vi "Periodic Tasks.vi"(8 "error in":errorcluster) -> ()   [LabVIEW 2013]
doc: "This VI runs in parallel to other tasks. It can contain as many user-defined periodic loops as you need. These can carry out PID or other sorts of timed response."
uses:
  PressureSensorAction.ctl
  <vilib>/Rock Robotics/SystemInterfaces/Utilities/FPGA_UtilitiesLED Source.ctl
  <vilib>/Rock Robotics/SystemInterfaces/Utilities/FPGA_UtilitiesLED State.ctl
  PassType.ctl
  PassState.ctl
  <vilib>/Rock Robotics/WPI/Compressor/WPI_CompressorGetSetRefNum.vi
  Robot Global Data.vi
panel:
  out "Pressure Sensor Iterations":i32
  out "Pressure Sensor Loop Time":u32
  out "Handler Iterations":i32
  in  "HalfDriveScalar":dbl=0.6
  out "Handler Skipped Data?":bool
  out "Main Loop Time":u32
  out "Handler Loop Time":u32
  out "Drive Loop Time":u32
  out "HandleInputElements":i32
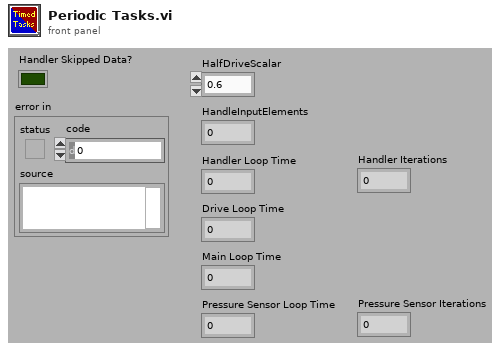
[diagram p1: front panel]
types:
  T1 = typedef "TeleopInstruction.ctl" = cluster{"cDriveLeft":dbl, "cDriveRight":dbl, "cAutoDistance":bool, "cHalfDrive":bool, "cStraightDrive":bool, "cReverseDrive":bool, "cSonicShifter":bool, "cRoller":dbl, "cCollector":dbl, "cServo":dbl, "cPass":bool, "cCatch":bool, "cCollectorWrap":bool, "cShooter":bool, "cClapperIn":bool, "cClapperOut":bool, "cFiringPneumatic":bool, "cKickerPneumatic":bool, "cRollerPneumatic":bool, "TeleopID":i32}
  T2 = typedef "DriveInstruction.ctl" = cluster{"DriveData":T3, "Subsystem":T4, "Action":T5}
  T3 = typedef "DriveData.ctl" = cluster{"cDriveLeft":dbl, "cDriveRight":dbl, "cHalfDrive":bool, "cStraightDrive":bool, "cReverseDrive":bool}
  T4 = typedef "QueueSubsystem.ctl" = enum16{"Drive", "SonicShifter", "Kicker", "FiringPneumatic", "RollerPneumatic", "Clapper", "RollerMotor", "CollectorMotor", "Servo", "ShooterWrapper", "CollectorWrapper", "CatcherWrapper", "AutoDistance", "PassWrapper"}
  T5 = typedef "TankDriveAction.ctl" = enum16{"Init", "LinearDrive", "SetValue", "Disable"}
  T6 = typedef "FPGA_UtilitiesLED State.ctl" = enum16{"Off", "On", "Toggle"}
  T7 = typedef "FPGA_UtilitiesLED Source.ctl" = enum16{"User LED", "FPGA LED"}
  T8 = typedef "PassType.ctl" = enum16{"Ground", "Elevated"}
  T9 = typedef "PassState.ctl" = enum16{"Pass", "Stop"}
  T10 = typedef "QueueInstruction.ctl" = cluster{"Data":variant, "Subsystem":T4, "Action":T11}
  T11 = typedef "QueueAction.ctl" = enum16{"Init", "SetValue", "Disable"}
  T12 = typedef "DoubleSolenoidAction.ctl" = enum16{"Init", "Middle", "In", "Out"}
  T13 = typedef "RollerAction.ctl" = enum16{"Init", "Off", "Forward", "Reverse"}
  T14 = typedef "CollectorWrapAction.ctl" = enum16{"PreCollect", "Collect", "Stop"}
  T15 = typedef "ServoAction.ctl" = enum16{"Init", "SetAngle", "GetAngle", "Lower", "Raise", "Disable"}
  T16 = typedef "ShooterWrapperAction.ctl" = enum16{"Init", "CollectorDown", "CollectorUp"}
  T17 = typedef "CatchAction.ctl" = enum16{"PreCatch", "Catch", "Stop"}
  T18 = typedef "PressureSensorAction.ctl" = enum16{"Init", "ReadValue", "Disable"}
  T19 = typedef "WPI_CompressorDevRef.ctl" = cluster{"DevStatus":errorcluster, "DigitalInputDevRef":T20, "RelayDevRef":T23}
  T20 = typedef "WPI_DigitalInputDevRef.ctl" = cluster{"DevStatus":errorcluster, "DIO Channel":T21, "Digital Module":T22}
  T21 = typedef "FPGA_DIOChannel.ctl" = enum8{"DIO 1", "DIO 2", "DIO 3", "DIO 4", "DIO 5", "DIO 6", "DIO 7", "DIO 8", "DIO 9", "DIO 10", "DIO 11", "DIO 12", "DIO 13", "DIO 14", "Invalid"}
  T22 = typedef "FPGA_TypedefDigitalModule.ctl" = enum16{"Digital Module 1", "Digital Module 2"}
  T23 = typedef "WPI_RelayDevRef.ctl" = cluster{"DevStatus":errorcluster, "Relay Channel":T24, "Digital Module":T22, "Relay Direction":T25}
  T24 = typedef "FPGA_DIORelayChannel.ctl" = enum8{"Relay 1", "Relay 2", "Relay 3", "Relay 4", "Relay 5", "Relay 6", "Relay 7", "Relay 8", "Invalid"}
  T25 = typedef "WPI_RelayDirection.ctl" = enum16{"Both directions", "Forward only", "Reverse only"}
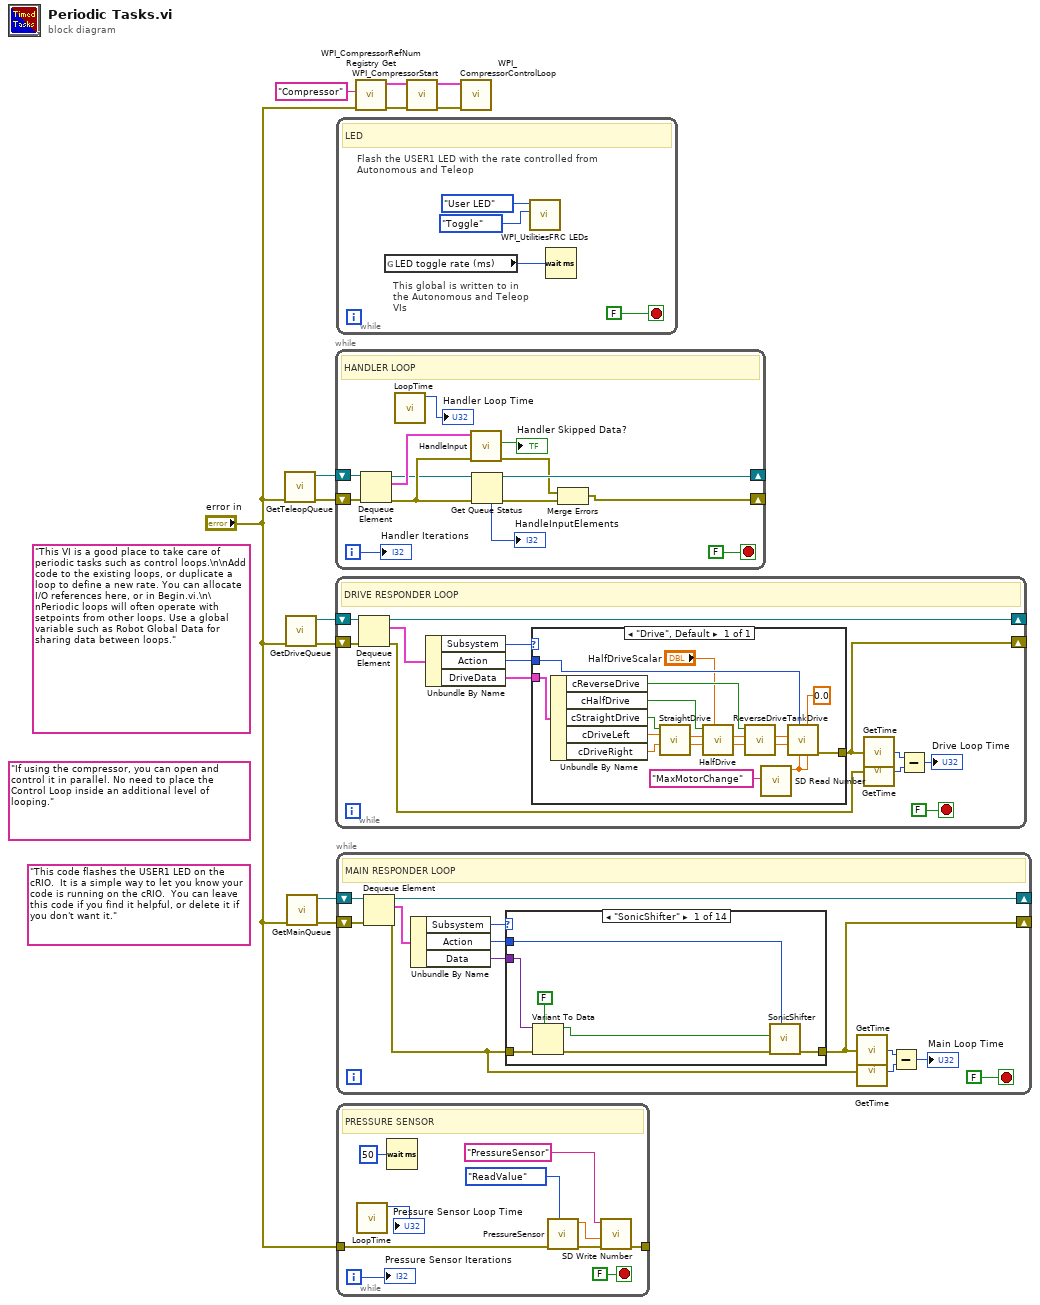
[diagram p0: block diagram]
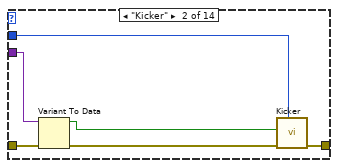
[diagram p2: hidden frame]
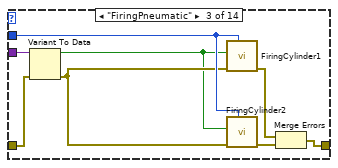
[diagram p3: hidden frame]
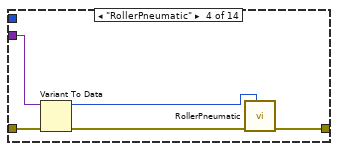
[diagram p4: hidden frame]
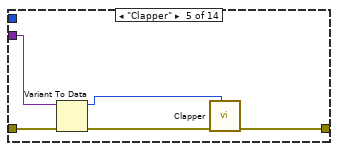
[diagram p5: hidden frame]
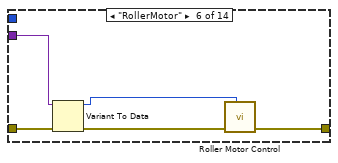
[diagram p6: hidden frame]
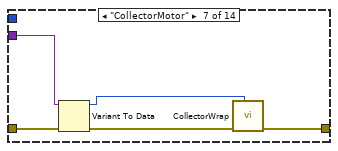
[diagram p7: hidden frame]
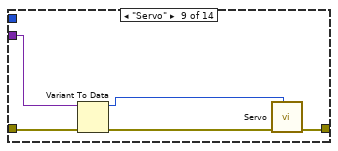
[diagram p9: hidden frame]
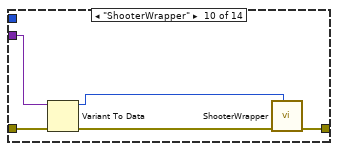
[diagram p10: hidden frame]
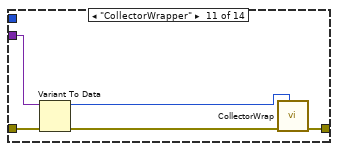
[diagram p11: hidden frame]
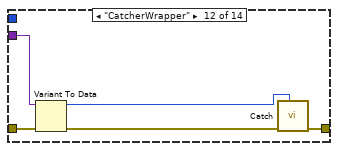
[diagram p12: hidden frame]
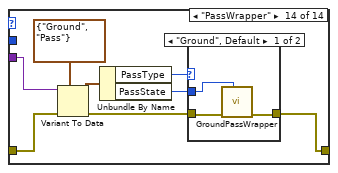
[diagram p14: hidden frame]
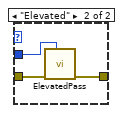
[diagram p15: hidden frame]
diagram:
  (unwired) "If using the compressor, you can open and control it in parallel. No need to place the Control Loop inside an additional level of looping."
  (unwired) "This code flashes the USER1 LED on the cRIO.  It is a simple way to let you know your code is running on the cRIO.  You can leave this code if you find it helpful, or delete it if you don't want it."
  (unwired) "This VI is a good place to take care of periodic tasks such as control loops.\n\nAdd code to the existing loops, or duplicate a loop to define a new rate. You can allocate I/O references here, or in Begin.vi.\n\nPeriodic loops will often operate with setpoints from other loops. Use a global variable such as Robot Global Data for sharing data between loops."
  n1 = call "GetTeleopQueue.vi"("error in (no error)"="error in") -> ("error out"=w6:errorcluster, "queue out"=w7:refnum<queue>)  [unwired: 9 in]
  n2 = call "GetDriveQueue.vi"("error in (no error)"="error in") -> ("error out"=w5:errorcluster, "queue out"=w4:refnum<queue>)  [unwired: 9 in]
  n3 = call "GetMainQueue.vi"("error in (no error)"="error in") -> ("error out"=w2:errorcluster, "queue out"=w3:refnum<queue>)  [unwired: 9 in]
  n4 = while {
    shift-right: [w17] -> _
    shift-left: w6 -> [w26]
    shift-right: [w24] -> _
    shift-left: w7 -> [w25]
    i -> [w13]
    stop <- FALSE stop-if-true
    # "HANDLER LOOP"
    n5 = Dequeue Element(queue=w25, error in (no error)=w26) -> (queue out=w20:refnum<queue>, element=w22:T1, error out=w21:errorcluster)  [unwired: 1 in, 1 out]
    n6 = call "LoopTime.vi"() -> ("LoopTime"=→"Handler Loop Time":u32)  [unwired: 11 in]
    n7 = call "HandleInput.vi"("error in (no error)"=w21, "TeleopInstruction"=w22) -> ("error out"=w18:errorcluster, "SkippedData?"=→"Handler Skipped Data?":bool)  [unwired: 7 in, 1 out]
    n8 = Get Queue Status(queue=w20, error in (no error)=w21) -> (queue out=w24:refnum<queue>, error out=w19:errorcluster, # elements in queue=→"HandleInputElements":i32)  [unwired: 1 in, 5 out]
    n9 = Merge Errors(w18, w19) -> (w17:errorcluster)
    "Handler Iterations" <- w13
  }
  n10 = while {
    shift-right: [w38] -> _
    shift-left: w4 -> [w39]
    shift-right: [w30] -> _
    shift-left: w5 -> [w37]
    stop <- FALSE stop-if-true
    # "DRIVE RESPONDER LOOP"
    n11 = Dequeue Element(queue=w39, error in (no error)=w37) -> (queue out=w38:refnum<queue>, element=w36:T2, error out=w31:errorcluster)  [unwired: 1 in, 1 out]
    n12 = Unbundle By Name(w36) -> ("Subsystem"=w35:T4, "Action"=w34:T5, "DriveData"=w33:T3)
    n13 = case shown="\"Drive\", Default" w35 {
      tunnel: w34 -> [w57]
      tunnel: w33 -> [w55]
      tunnel: [w43] -> w30
      frame "Drive", Default {
        n14 = Unbundle By Name(w55) -> ("cReverseDrive"=w46:bool, "cHalfDrive"=w45:bool, "cStraightDrive"=w44:bool, "cDriveLeft"=w54:dbl, "cDriveRight"=w53:dbl)
        n15 = call "StraightDrive.vi"("RightDrive in"=w53, "LeftDrive in"=w54, "StraightDrive"=w44) -> ("RightDrive out"=w51:dbl, "LeftDrive out"=w52:dbl)  [unwired: 7 in]
        n16 = call "HalfDrive.vi"("Scaler"="HalfDriveScalar", "RightDrive in"=w51, "LeftDrive in"=w52, "HalfDrive"=w45) -> ("RightDrive out"=w49:dbl, "LeftDrive out"=w50:dbl)  [unwired: 6 in]
        n17 = call "ReverseDrive.vi"("Right"=w49, "Left"=w50, "cReverseDrive"=w46) -> ("Right"=w47:dbl, "Left"=w48:dbl)  [unwired: 7 in]
        n18 = call <vilib>:"SD Read Number.vi"("Name"="MaxMotorChange") -> ("Numeric"=w40:dbl)  [unwired: 8 in, 2 out]
        n19 = call "TankDrive.vi"("MaxMotorChangeForward"=w40, "Cutoff"=0.0, "MaxMotorChangeBackward"=w40, "DriveAction"=w57, "RightDesired"=w47, "LeftDesired"=w48) -> ("error out"=w43:errorcluster)  [unwired: 4 in, 1 out]
      }
    }
    n20 = call "GetTime.vi"("error in"=w30) -> ("Time"=w28:u32)
    n21 = call "GetTime.vi"("error in"=w31) -> ("Time"=w29:u32)
    n22 = Subtract(x=w28, y=w29) -> (x-y=→"Drive Loop Time":u32)
  }
  n23 = while {
    stop <- FALSE stop-if-true
    # "This global is written to in the Autonomous and Teleop VIs"
    # "Flash the USER1 LED with the rate controlled from Autonomous and Teleop"
    # "LED"
    n24 = global read "Robot Global Data.vi" "LED toggle rate (ms)"() -> (w58:u32)
    n25 = call <vilib>:"WPI_UtilitiesFRC LEDs.vi"("State"=FPGA_UtilitiesLED_State."Toggle", "LED Type"=FPGA_UtilitiesLED_Source."User LED") -> ()  [unwired: 1 in, 9 out]
    n26 = Wait (ms)(milliseconds to wait=w58) -> ()  [unwired: 1 out]
  }
  n27 = while {
    shift-right: [w72] -> _
    shift-left: w3 -> [w73]
    shift-right: [w66] -> _
    shift-left: w2 -> [w74]
    stop <- FALSE stop-if-true
    # "MAIN RESPONDER LOOP"
    n28 = Dequeue Element(queue=w73, error in (no error)=w74) -> (queue out=w72:refnum<queue>, element=w71:T10, error out=w62:errorcluster)  [unwired: 1 in, 1 out]
    n29 = Unbundle By Name(w71) -> ("Subsystem"=w70:T4, "Action"=w69:T11, "Data"=w68:variant)
    n30 = case shown="\"SonicShifter\"" w70 {
      tunnel: [w77 w87 w92 w100 w105 w110 w112 w116 w121 w126 w131 w136 _ w144] -> w66
      tunnel: w62 -> [w79 w86 w90 w97 w104 w108 w115 w116 w119 w125 w130 w135 _ w141]
      tunnel: w69 -> [w81 w82 w94 _ _ _ _ _ _ _ _ _ _ _]
      tunnel: w68 -> [w80 w84 w95 w99 w102 w109 w114 _ w118 w123 w127 w132 _ w143]
      frame "SonicShifter" {
        n31 = Variant To Data(error in=w79, type=FALSE, Variant=w80) -> (data=w76:bool, error out=w78:errorcluster)
        n32 = call "SonicShifter.vi"("Action"=w81, "error in (no error)"=w78, "Actuate?"=w76) -> ("error out"=w77:errorcluster)  [unwired: 8 in]
      }
      frame "Kicker" {
        n33 = Variant To Data(error in=w86, Variant=w84) -> (data=w83:bool, error out=w85:errorcluster)  [unwired: 1 in]
        n34 = call "Kicker.vi"("Action"=w82, "error in (no error)"=w85, "Actuate?"=w83) -> ("error out"=w87:errorcluster)  [unwired: 8 in]
      }
      frame "FiringPneumatic" {
        n35 = Variant To Data(error in=w90, Variant=w95) -> (data=w88:bool, error out=w89:errorcluster)  [unwired: 1 in]
        n36 = call "FiringCylinder1.vi"("Action"=w94, "error in (no error)"=w89, "Actuate?"=w88) -> ("error out"=w91:errorcluster)  [unwired: 8 in]
        n37 = call "FiringCylinder2.vi"("Action"=w94, "error in (no error)"=w89, "Actuate?"=w88) -> ("error out"=w93:errorcluster)  [unwired: 8 in]
        n38 = Merge Errors(w91, w93) -> (w92:errorcluster)
      }
      frame "RollerPneumatic" {
        n39 = Variant To Data(error in=w97, Variant=w99) -> (data=w98:T12, error out=w96:errorcluster)  [unwired: 1 in]
        n40 = call "RollerPneumatic.vi"("State"=w98, "Error in"=w96) -> ("Error out"=w100:errorcluster)  [unwired: 9 in]
      }
      frame "Clapper" {
        n41 = Variant To Data(error in=w104, Variant=w102) -> (data=w101:T12, error out=w103:errorcluster)  [unwired: 1 in]
        n42 = call "Clapper.vi"("State"=w101, "Error in"=w103) -> ("Error out"=w105:errorcluster)  [unwired: 9 in]
      }
      frame "RollerMotor" {
        n43 = Variant To Data(error in=w108, Variant=w109) -> (data=w106:T13, error out=w107:errorcluster)  [unwired: 1 in]
        n44 = call "Roller Motor Control.vi"("Action"=w106, "Error in"=w107) -> ("Error out"=w110:errorcluster)  [unwired: 9 in]
      }
      frame "CollectorMotor" {
        n45 = Variant To Data(error in=w115, Variant=w114) -> (data=w111:T14, error out=w113:errorcluster)  [unwired: 1 in]
        n46 = call "CollectorWrap.vi"("Action"=w111, "error in"=w113) -> ("error out"=w112:errorcluster)  [unwired: 8 in, 1 out]
      }
      frame "Drive" {
        # "\"Should\" be handled in drive loop"
      }
      frame "Servo" {
        n47 = Variant To Data(error in=w119, Variant=w118) -> (data=w117:T15, error out=w120:errorcluster)  [unwired: 1 in]
        n48 = call "Servo.vi"("Action"=w117, "error in (no error)"=w120) -> ("error out"=w121:errorcluster)  [unwired: 8 in, 1 out]
      }
      frame "ShooterWrapper" {
        n49 = Variant To Data(error in=w125, Variant=w123) -> (data=w122:T16, error out=w124:errorcluster)  [unwired: 1 in]
        n50 = call "ShooterWrapper.vi"("Action"=w122, "error in"=w124) -> ("error out"=w126:errorcluster)  [unwired: 8 in]
      }
      frame "CollectorWrapper" {
        n51 = Variant To Data(error in=w130, Variant=w127) -> (data=w128:T14, error out=w129:errorcluster)  [unwired: 1 in]
        n52 = call "CollectorWrap.vi"("Action"=w128, "error in"=w129) -> ("error out"=w131:errorcluster)  [unwired: 8 in, 1 out]
      }
      frame "CatcherWrapper" {
        n53 = Variant To Data(error in=w135, Variant=w132) -> (data=w133:T17, error out=w134:errorcluster)  [unwired: 1 in]
        n54 = call "Catch.vi"("Action"=w133, "error in (no error)"=w134) -> ("error out"=w136:errorcluster)  [unwired: 9 in]
      }
      frame "AutoDistance" {
      }
      frame "PassWrapper" {
        n55 = Variant To Data(error in=w141, type=cluster{"PassType":T8, "PassState":T9} {"PassType"=enum."Ground", "PassState"=enum."Pass"}, Variant=w143) -> (data=w139:cluster{"PassType":T8, "PassState":T9}, error out=w140:errorcluster)
        n56 = Unbundle By Name(w139) -> ("PassType"=w138:T8, "PassState"=w137:T9)
        n57 = case shown="\"Ground\", Default" w138 {
          tunnel: [w147 w149] -> w144
          tunnel: w140 -> [w146 w150]
          tunnel: w137 -> [w145 w148]
          frame "Ground", Default {
            n58 = call "GroundPassWrapper.vi"("State"=w145, "error in"=w146) -> ("error out"=w147:errorcluster)  [unwired: 9 in]
          }
          frame "Elevated" {
            n59 = call "ElevatedPass.vi"("PassState"=w148, "error in (no error)"=w150) -> ("error out"=w149:errorcluster)  [unwired: 9 in]
          }
        }
      }
    }
    n60 = call "GetTime.vi"("error in"=w66) -> ("Time"=w65:u32)
    n61 = call "GetTime.vi"("error in"=w62) -> ("Time"=w64:u32)
    n62 = Subtract(x=w65, y=w64) -> (x-y=→"Main Loop Time":u32)
  }
  n63 = while {
    tunnel: "error in" -> [w159]
    tunnel: [w156] -> _
    i -> [w152]
    stop <- FALSE stop-if-true
    # "PRESSURE SENSOR"
    n64 = call "LoopTime.vi"() -> ("LoopTime"=→"Pressure Sensor Loop Time":u32)  [unwired: 11 in]
    n65 = Wait (ms)(milliseconds to wait=u32 50) -> ()  [unwired: 1 out]
    n66 = call "PressureSensor.vi"("Action"=PressureSensorAction."ReadValue", "error in (no error)"=w159) -> ("error out"=w157:errorcluster, "Pressure"=w155:dbl)  [unwired: 8 in]
    n67 = call <vilib>:"SD Write Number.vi"("error in"=w157, "Numeric"=w155, "Name"="PressureSensor") -> ("error out"=w156:errorcluster)  [unwired: 7 in, 1 out]
    "Pressure Sensor Iterations" <- w152
  }
  n68 = call <vilib>:"WPI_CompressorRefNum Registry Get.vi"("error in (no error)"="error in", "refnum name"="Compressor") -> ("error out"=w11:errorcluster, "CompressorDevRef"=w10:T19)  [unwired: 8 in]
  n69 = call <vilib>:"WPI_CompressorStart.vi"("error in (no error)"=w11, "CompressorDevRef"=w10) -> ("error out"=w9:errorcluster, "CompressorDevRef"=w8:T19)  [unwired: 8 in]
  n70 = call <vilib>:"WPI_CompressorControlLoop.vi"("error in (no error)"=w9, "CompressorDevRef"=w8) -> ()  [unwired: 10 in]
